vi "niLvFpga_ReadBigControl_cRIO-9041.vi"(0 "session in":u32, 7 "Address":u32, 9 "repeat":u32, 11 "error in":errorcluster) -> (4 "session out":u32, 8 "data out":u32[](array[numeric]), 15 "error out":errorcluster)   [LabVIEW 2020]
uses:
  NiFpgaLv.dll
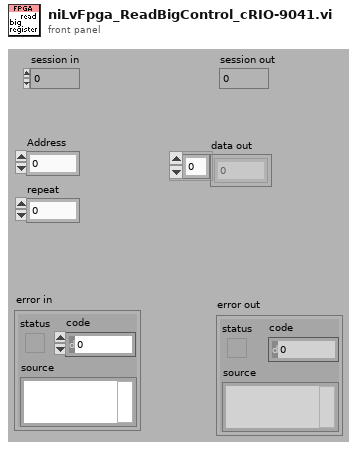
[diagram p1: front panel]
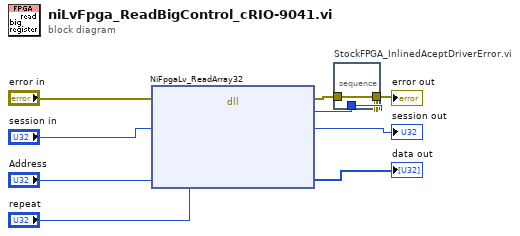
[diagram p0: block diagram]
diagram:
  n1 = dll-call lib="NiFpgaLv.*" fn="NiFpgaLv_ReadArray32" label="niLvFpgaReadBigControl"(error in="error in", "sessionID"="session in", "offset"="Address", "repeat"="repeat") -> (error out=w5:errorcluster, "status"=w4:i32, "sessionID"=→"session out":u32, "Data"=→"data out":u32[])  [unwired: 5 in, 1 out]
  n2 = stacked-sequence "StockFPGA_InlinedAceptDriverError.vi" {
    tunnel: w5 -> [w10]
    tunnel: w4 -> [w12]
    tunnel: [w11] -> w3
    frame #0 {
      n3 = case shown="Default" w12 {
        selector: w12 -> [_ w14]
        tunnel: [w13 w16] -> w11
        tunnel: w10 -> [w13 w17]
        frame 0 {
        }
        frame Default {
          n4 = Greater Than 0?(x=w14) -> (x > 0?=w15:bool)
          n5 = call <vilib>:"Error Cluster From Error Code.vi"("is warning? (False)"=w15, "error in (no error)"=w17, "error code (0)"=w14) -> ("error out"=w16:errorcluster)  [unwired: 6 in]
        }
      }
    }
  }
  "error out" <- w3
